vi "Read_Multiple_ERD.vi"(0 "session in":refnum<k35>, 5 "Board":u8, 7 "dst":i64, 9 "Read ERD":i64[](array[numeric]) format="%x", 11 "error out":errorcluster) -> (4 "session out":refnum<k35>, 8 "Multiple Read":T1 {"ERD Number" format="%x"}, 15 "error IO":errorcluster)   [LabVIEW 2021]
uses:
  Controles/Multiple_Read_ERD.ctl
  Controles/Read_ERD.ctl
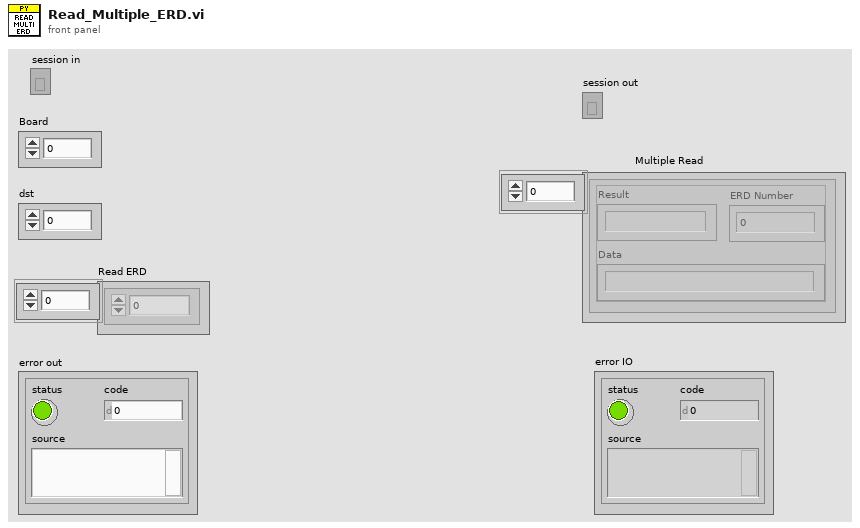
[diagram p1: front panel]
types:
  T1 = typedef "Multiple_Read_ERD.ctl" = T2[]
  T2 = typedef "Read_ERD.ctl" = cluster{"Result":string, "ERD Number":i64, "Data":string}
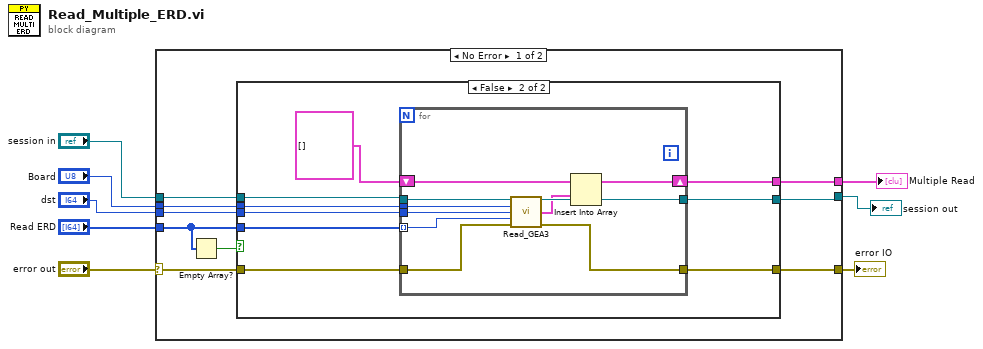
[diagram p0: block diagram]
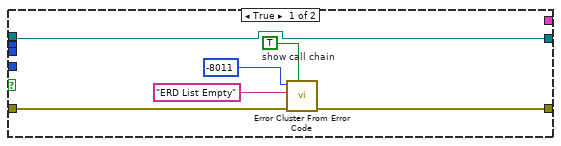
[diagram p2: hidden frame]
diagram:
  n1 = case shown="No Error" "error out" {
    selector: "error out" -> [w14 w44]
    tunnel: "Read ERD" -> [w12 _]
    tunnel: "session in" -> [w17 w43]
    tunnel: "Board" -> [w16 _]
    tunnel: "dst" -> [w15 _]
    tunnel: [w11 w44] -> w2
    tunnel: [w10 _] -> w3
    tunnel: [w9 w43] -> w1
    frame No Error {
      n2 = Empty Array?(array=w12) -> (empty?=w13:bool)
      n3 = case shown="False" w13 {
        tunnel: w12 -> [_ w32]
        tunnel: w17 -> [w18 w30]
        tunnel: w16 -> [_ w29]
        tunnel: w15 -> [_ w28]
        tunnel: w14 -> [w20 w27]
        tunnel: [w19 w26] -> w11
        tunnel: [_ w25] -> w10
        tunnel: [w18 w24] -> w9
        frame True {
          w23 = TRUE  # show call chain
          n4 = call <vilib>:"Error Cluster From Error Code.vi"("show call chain? (False)"=w23, "error in (no error)"=w20, "error message (\"\")"="ERD List Empty" ("error message (\"\")"), "error code (0)"=-8011) -> ("error out"=w19:errorcluster)  [unwired: 5 in]
        }
        frame False {
          n5 = for {
            tunnel: w29 -> [w41]
            tunnel: w28 -> [w40]
            tunnel: w30 -> [w42]
            tunnel: [w39] -> w24
            tunnel: [w38] -> w26
            tunnel: w32 -> [w37] mode=indexing
            shift-right: [w34] -> w25
            shift-left: T1 [] ("Multiple Read") -> [w35]
            tunnel: w27 -> [w33]
            n6 = call "Read_GEA3.vi"("session in"=w42, "board"=w41, "dst"=w40, "ERD"=w37, "error in (no error)"=w33) -> ("session out"=w39:refnum<k35>, "Read ERD"=w36:T2, "error out"=w38:errorcluster)  [unwired: 8 in]
            n7 = Insert Into Array(array=w35, new element=w36) -> (w34:T1)  [unwired: 1 in]
          }
        }
      }
    }
    frame Error {
    }
  }
  "Multiple Read" <- w3
  "error IO" <- w2
  "session out" <- w1
